vi "laserDiagnose_III.vi"(0 "405 Port":refnum<visa-resource-name>, 5 "532 Port in":refnum<visa-resource-name>, 7 "660 Port 3":refnum<visa-resource-name>, 11 "error in (no error)":errorcluster, 12 "ms to wait (50)":u32=50) -> (4 "Powers":T3, 6 "Currents":T1, 8 "Temperatures":T2, 10 "Overtemp":bool, 15 "error out":errorcluster)   [LabVIEW 2011]
panel:
  out "660 Port Out":refnum<visa-resource-name>
  out "532 Port Out":refnum<visa-resource-name>
  out "405 Port Out":refnum<visa-resource-name>
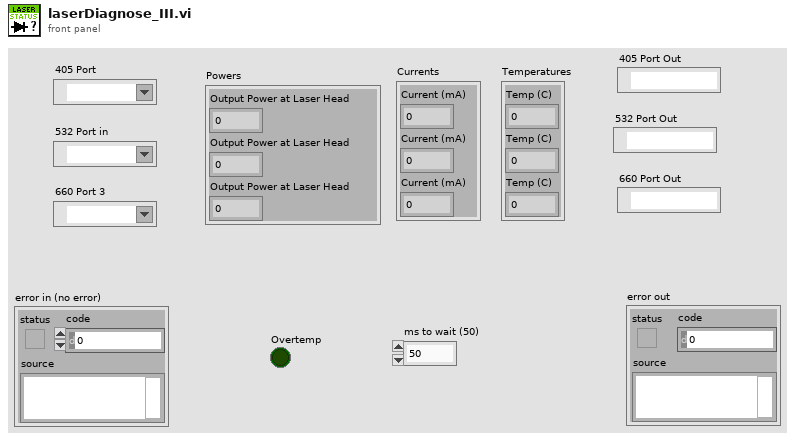
[diagram p1: front panel]
types:
  T1 = cluster{"Current (mA)":dbl, "Current (mA)":dbl, "Current (mA)":dbl}
  T2 = cluster{"Temp (C)":dbl, "Temp (C)":dbl, "Temp (C)":dbl}
  T3 = cluster{"Output Power at Laser Head":dbl, "Output Power at Laser Head":dbl, "Output Power at Laser Head":dbl}
  T4 = cluster{"Current, mA":dbl, "Current, mA":dbl, "Current, mA":dbl}
  T5 = cluster{"Power, mW":dbl, "Power, mW":dbl, "Power, mW":dbl}
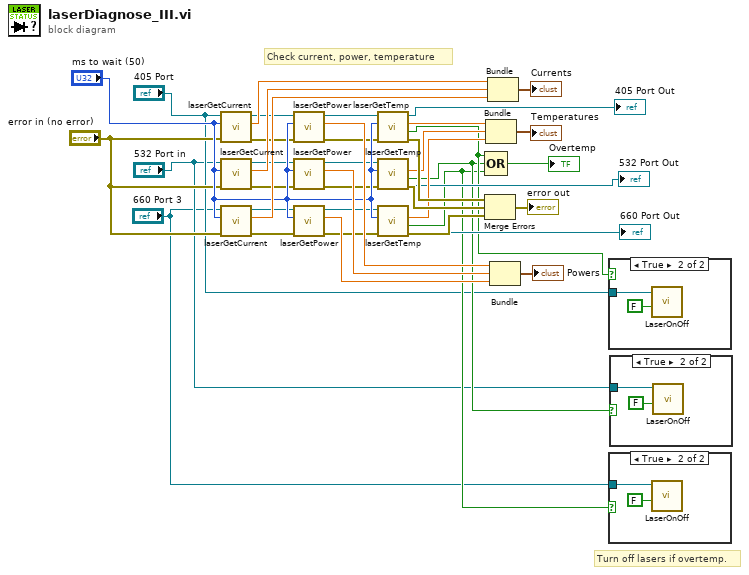
[diagram p0: block diagram]
diagram:
  # "Check current, power, temperature"
  # "Turn off lasers if overtemp."
  n1 = call "laserGetCurrent.vi"("error in (no error)"="error in (no error)", "ms to wait (5)"="ms to wait (50)", "VISA resource name"="405 Port") -> ("error out"=w17:errorcluster, "Current, mA"=w25:dbl, "VISA resource name out"=w11:refnum<visa-resource-name>)  [unwired: 6 in]
  n2 = call "laserGetCurrent.vi"("error in (no error)"="error in (no error)", "ms to wait (5)"="ms to wait (50)", "VISA resource name"="532 Port in") -> ("error out"=w19:errorcluster, "Current, mA"=w26:dbl, "VISA resource name out"=w13:refnum<visa-resource-name>)  [unwired: 6 in]
  n3 = call "laserGetCurrent.vi"("error in (no error)"="error in (no error)", "ms to wait (5)"="ms to wait (50)", "VISA resource name"="660 Port 3") -> ("error out"=w22:errorcluster, "Current, mA"=w27:dbl, "VISA resource name out"=w15:refnum<visa-resource-name>)  [unwired: 6 in]
  n4 = call "laserGetPower.vi"("error in (no error)"=w17, "ms to wait (5)"="ms to wait (50)", "VISA resource name"=w11) -> ("error out"=w18:errorcluster, "Power, mW"=w33:dbl, "VISA resource name out"=w12:refnum<visa-resource-name>)  [unwired: 6 in]
  n5 = call "laserGetPower.vi"("error in (no error)"=w19, "ms to wait (5)"="ms to wait (50)", "VISA resource name"=w13) -> ("error out"=w20:errorcluster, "Power, mW"=w34:dbl, "VISA resource name out"=w14:refnum<visa-resource-name>)  [unwired: 6 in]
  n6 = call "laserGetPower.vi"("error in (no error)"=w22, "ms to wait (5)"="ms to wait (50)", "VISA resource name"=w15) -> ("error out"=w21:errorcluster, "Power, mW"=w35:dbl, "VISA resource name out"=w16:refnum<visa-resource-name>)  [unwired: 6 in]
  n7 = call "laserGetTemp.vi"("error in (no error)"=w18, "milliseconds to wait"="ms to wait (50)", "VISA resource name"=w12) -> ("error out"=w37:errorcluster, "Overtemp"=w6:bool, "Temp (C)"=w29:dbl, "VISA resource name out"=→"405 Port Out":refnum<visa-resource-name>)  [unwired: 5 in]
  n8 = call "laserGetTemp.vi"("error in (no error)"=w20, "milliseconds to wait"="ms to wait (50)", "VISA resource name"=w14) -> ("error out"=w38:errorcluster, "Overtemp"=w5:bool, "Temp (C)"=w30:dbl, "VISA resource name out"=→"532 Port Out":refnum<visa-resource-name>)  [unwired: 5 in]
  n9 = call "laserGetTemp.vi"("error in (no error)"=w21, "milliseconds to wait"="ms to wait (50)", "VISA resource name"=w16) -> ("error out"=w39:errorcluster, "Overtemp"=w4:bool, "Temp (C)"=w31:dbl, "VISA resource name out"=→"660 Port Out":refnum<visa-resource-name>)  [unwired: 5 in]
  n10 = Compound Arithmetic op=OR(w6, w5, w4) -> (→"Overtemp":bool)
  n11 = Merge Errors(w37, w38, w39) -> (→"error out":errorcluster)
  n12 = Bundle("Temp (C)"=w29, "Temp (C)"=w30, "Temp (C)"=w31) -> (→"Temperatures":T2)  [unwired: 1 in]
  n13 = Bundle("Current, mA"=w25, "Current, mA"=w26, "Current, mA"=w27) -> (→"Currents":T4)  [unwired: 1 in]
  n14 = Bundle("Power, mW"=w33, "Power, mW"=w34, "Power, mW"=w35) -> (→"Powers":T5)  [unwired: 1 in]
  n15 = case shown="True" w6 {
    tunnel: "405 Port" -> [_ w42]
    frame False {
    }
    frame True {
      n16 = call "LaserOnOff.vi"("Emission (F = OFF)"=FALSE ("405 Emission (T = ON)"), "VISA Refnum in"=w42) -> ()  [unwired: 7 in, 3 out]
    }
  }
  n17 = case shown="True" w4 {
    tunnel: "660 Port 3" -> [_ w44]
    frame False {
    }
    frame True {
      n18 = call "LaserOnOff.vi"("Emission (F = OFF)"=FALSE ("405 Emission (T = ON)"), "VISA Refnum in"=w44) -> ()  [unwired: 7 in, 3 out]
    }
  }
  n19 = case shown="True" w5 {
    tunnel: "532 Port in" -> [_ w46]
    frame False {
    }
    frame True {
      n20 = call "LaserOnOff.vi"("Emission (F = OFF)"=FALSE ("405 Emission (T = ON)"), "VISA Refnum in"=w46) -> ()  [unwired: 7 in, 3 out]
    }
  }
